vi "Device Deactivate (Emergency).vi"(8 "error in (no error)":errorcluster, 11 "IED in":refnum<class "IED.lvclass">) -> (0 "error out":errorcluster, 3 "IED out":refnum<class "IED.lvclass">)   [LabVIEW 2015, in "IED Actor.lvlib" / "IED.lvclass"]
uses:
  IED.lvclass
  IED.lvclass/IED.ctl
  <vilib>/ActorFramework/Actor/Actor.lvclass/Actor.ctl
  SCADA Core/SCADA Emergency Messages/Emergency Fatal Error Msg/Emergency Fatal Error Msg.lvclass/Emergency Fatal Error Msg.ctl
  <vilib>/ActorFramework/Message Enqueuer/Message Enqueuer.lvclass/Message Enqueuer.ctl
  <vilib>/ActorFramework/Message Enqueuer/Enqueue.vi
  <vilib>/ActorFramework/Message Priority Queue/Priority Enqueue.vi
  SCADA Core/SCADA Emergency Messages/Emergency Fatal Error Msg/Emergency Fatal Error Msg.lvclass
  <vilib>/Modbus/master/Modbus Master.lvclass
  <vilib>/ActorFramework/Actor/Actor.lvclass
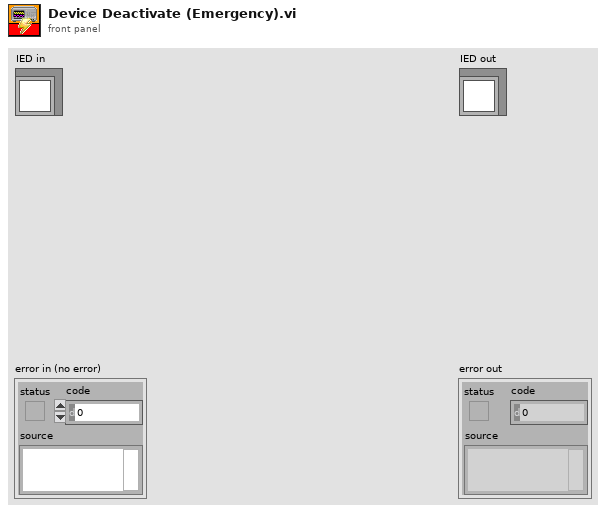
[diagram p1: front panel]
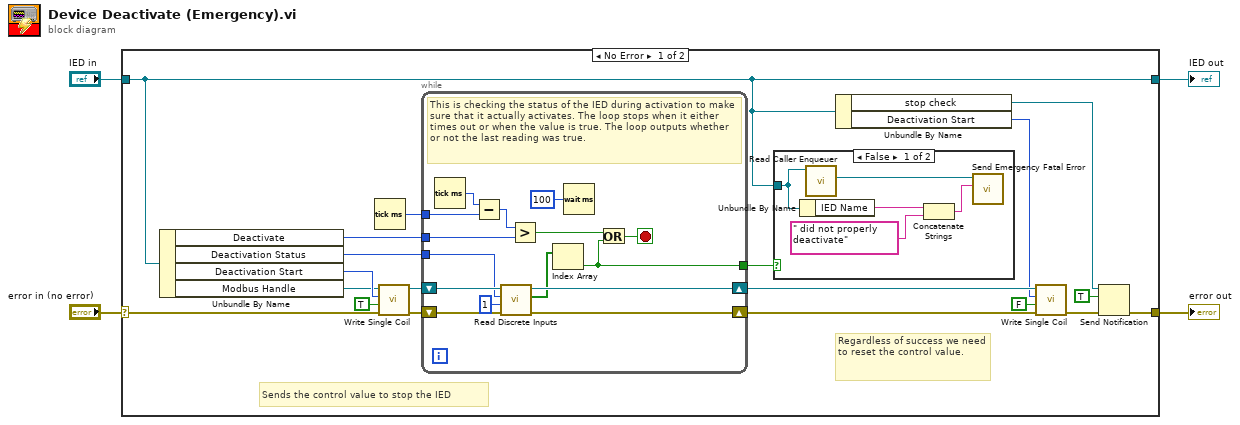
[diagram p0: block diagram]
diagram:
  n1 = case shown="No Error" "error in (no error)" {
    selector: "error in (no error)" -> [w7 w45]
    tunnel: [w12 w45] -> w3
    tunnel: [w9 w44] -> w1
    tunnel: "IED in" -> [w9 w44]
    frame No Error {
      # "Regardless of success we need to reset the control value."
      # "Sends the control value to stop the IED"
      n2 = Unbundle By Name(w9) -> ("Deactivate"=w17:u32, "Deactivation Status"=w18:u16, "Deactivation Start"=w22:u16, "Modbus Handle"=w6:refnum<class "Modbus Master.lvclass">)
      n3 = Tick Count (ms)() -> (millisecond timer value=w23:u32)
      n4 = call-dynamic "Write Single Coil.vi"("error in (no error)"=w7, "coil value"=TRUE, "address"=w22, "Modbus master in"=w6) -> ("error out"=w19:errorcluster, "Modbus master out"=w20:refnum<class "Modbus Master.lvclass">)  [unwired: 6 in]
      n5 = while {
        tunnel: w23 -> [w41]
        tunnel: w17 -> [w39]
        tunnel: w18 -> [w35]
        shift-right: [w29] -> w16
        shift-left: w19 -> [w34]
        tunnel: [w30] -> w8
        shift-right: [w32] -> w15
        shift-left: w20 -> [w36]
        stop <- w37 stop-if-true
        # "This is checking the status of the IED during activation to make sure that it actually activates. The loop stops when it either times out or when the value is true. The loop outputs whether or not the last reading was true."
        n6 = Tick Count (ms)() -> (millisecond timer value=w42:u32)
        n7 = Subtract(x=w42, y=w41) -> (x-y=w40:u32)
        n8 = call-dynamic "Read Discrete Inputs.vi"("error in (no error)"=w34, "number of discrete inputs"=u16 1 ("number of coils"), "starting address"=w35, "Modbus master in"=w36) -> ("error out"=w29:errorcluster, "discrete input values"=w31:bool[], "Modbus master out"=w32:refnum<class "Modbus Master.lvclass">)  [unwired: 5 in]
        n9 = Greater?(x=w40, y=w39) -> (0:w38:bool)
        n10 = Index Array(array=w31) -> (element=w30:bool)  [unwired: 1 in]
        n11 = Wait (ms)(milliseconds to wait=u32 100) -> ()  [unwired: 1 out]
        n12 = Or(x=w38, y=w30) -> (x .or. y?=w37:bool)
      }
      n13 = case shown="False" w8 {
        tunnel: w9 -> [w28 _]
        frame False {
          n14 = Unbundle By Name(w28) -> ("IED Name"=w26:string)
          n15 = call <vilib>:"Read Caller Enqueuer.vi"("Actor"=w28) -> ("Caller Enqueuer"=w27:refnum<class "Message Enqueuer.lvclass">)  [unwired: 10 in]
          n16 = Concatenate Strings(w26, " did not properly deactivate" ("string")) -> (w24:string)
          n17 = call "Send Emergency Fatal Error.vi"("Error"=w24, "Message Enqueuer"=w27) -> ()  [unwired: 8 in, 2 out]
        }
        frame True {
        }
      }
      n18 = Unbundle By Name(w9) -> ("stop check"=w11:refnum<notifier>, "Deactivation Start"=w14:u16)
      n19 = call-dynamic "Write Single Coil.vi"("error in (no error)"=w16, "coil value"=FALSE, "address"=w14, "Modbus master in"=w15) -> ("error out"=w5:errorcluster)  [unwired: 6 in, 1 out]
      n20 = Send Notification(notification=TRUE, notifier=w11, error in (no error)=w5) -> (error out=w12:errorcluster)  [unwired: 1 out]
    }
    frame Error {
    }
  }
  "error out" <- w3
  "IED out" <- w1
